vi "Target Motor Command.vi"(8 "Motor Instructions":T1, 11 "Motion Handle":refnum<k21>="nism://NI-PXIe8880-2F1836AB/AKM74L Motor") -> ()   [LabVIEW 2018, in "COBRA Kollmorgen Motor IO Library.lvlib"]
uses:
  COBRA Kollmorgen Motor IO Library.lvlib
  Target Motor Instructions.ctl
  Target Motor Command Options.ctl
  <resource>/objmgr/nimcai.rc
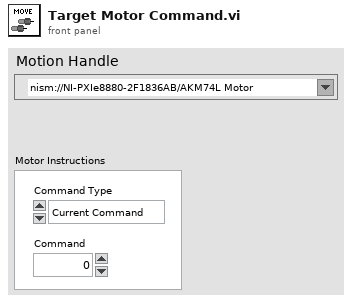
[diagram p1: front panel]
types:
  T1 = typedef "COBRA Kollmorgen Motor IO Library.lvlib/Target Motor Instructions.ctl" = cluster{"Command Type":T2, "Command":dbl}
  T2 = typedef "COBRA Kollmorgen Motor IO Library.lvlib/Target Motor Command Options.ctl" = enum16{"Current Command", "Velocity Command"}
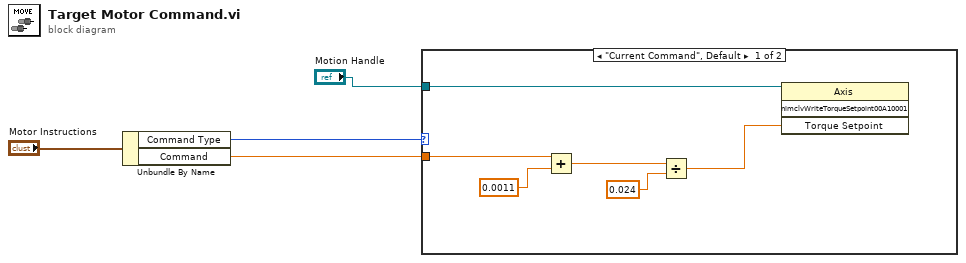
[diagram p0: block diagram]
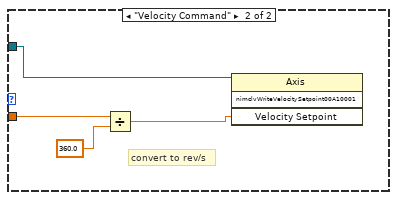
[diagram p2: hidden frame]
diagram:
  n1 = Unbundle By Name("Motor Instructions") -> ("Command Type"=w3:T2, "Command"=w2:dbl)
  n2 = case shown="\"Current Command\", Default" w3 {
    tunnel: "Motion Handle" -> [w10 w14]
    tunnel: w2 -> [w9 w13]
    frame "Current Command", Default {
      n3 = Add(x=w9, y=0.0011) -> (x+y=w7:dbl)
      n4 = Divide(x=w7, y=0.024) -> (x/y=w6:dbl)
      n5 = invoke on="Invoke Node" class="Axis" method="nimclvWriteTorqueSetpoint00A10001"(reference=w10, "Torque Setpoint"=w6) -> ()  [unwired: 2 in, 4 out]
    }
    frame "Velocity Command" {
      # "convert to rev/s"
      n6 = Divide(x=w13, y=360.0) -> (x/y=w11:dbl)
      n7 = invoke on="Invoke Node" class="Axis" method="nimclvWriteVelocitySetpoint00A10001"(reference=w14, "Velocity Setpoint"=w11) -> ()  [unwired: 2 in, 4 out]
    }
  }
